vi "Find Workspace.vi"(8 "Error In":errorcluster, 10 "Control In":T2={"I-O.lvclass"=refnum, "Motion.lvclass"=refnum, "Dispenser.lvclass"=refnum}, 11 "Workspace In":refnum<class "Fixture.lvclass">) -> (0 "Error Out":errorcluster, 1 "Workspace Out":T1, 2 "Control Out":T2, 3 "Workspace Out":refnum<class "Fixture.lvclass">)   [LabVIEW 2016, in "Fixture.lvclass"]
uses:
  Fixture.lvclass
  Controller/Controllers.ctl
  Controller/I-O/I-O.lvclass
  Controller/Motion/A3200/A3200.lvclass
  Controller/Dispenser/Dispenser.lvclass
  Controller/Motion/Motion.lvclass
  Workspace.ctl
  Fixture.lvclass/Fixture.ctl
  Controller/Controller.lvclass
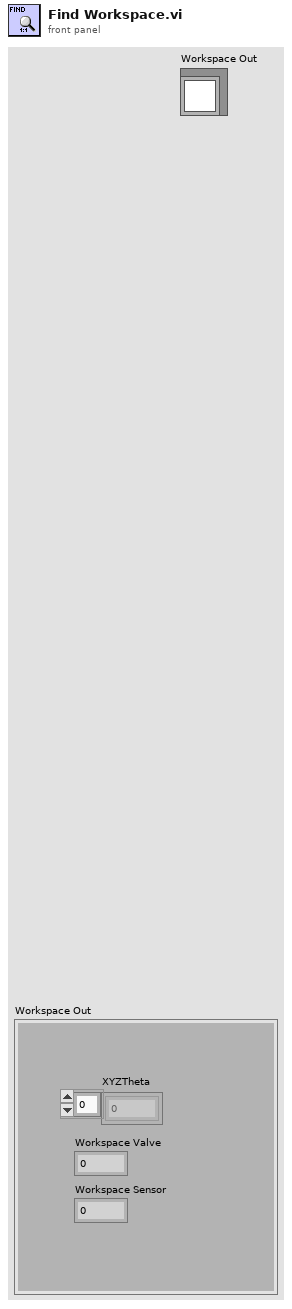
[diagram p1: front panel]
types:
  T1 = typedef "Fixture.lvclass/Workspace.ctl" = cluster{"XYZTheta":dbl[], "Workspace Valve":i32, "Workspace Sensor":i32}
  T2 = typedef "Controller.lvclass/Controllers.ctl" = cluster{"I-O.lvclass":refnum<class "I-O.lvclass">, "Motion.lvclass":refnum<class "Motion.lvclass">, "Dispenser.lvclass":refnum<class "Dispenser.lvclass">}
  T3 = typedef "I-O.lvclass/Pin Map.ctl" = cluster{"Region Valves":i32[], "Extra Valves":dbl[][][], "Tool Primary Valve":i32, "Tool Secondary Valve":i32, "Region Sensors":i32[], "Extra Sensors":dbl[][][], "Tool Primary Sensor":dbl, "Tool Secondary Sensor":dbl, "Compression Sensor":dbl, "5V":i32}
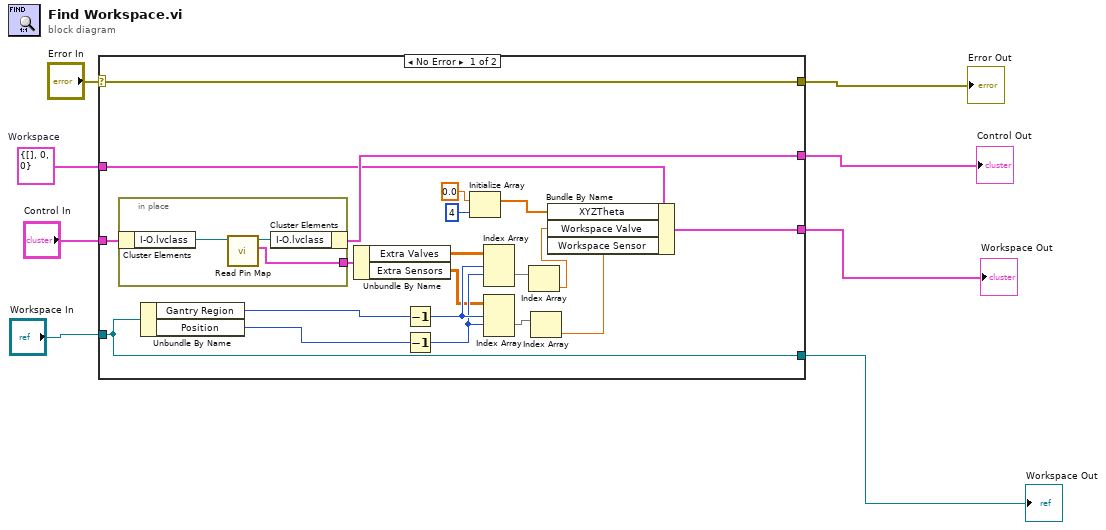
[diagram p0: block diagram]
diagram:
  w4 = T1 {"XYZTheta"=[], "Workspace Valve"=0, "Workspace Sensor"=0}  # Workspace
  n1 = case shown="No Error" "Error In" {
    selector: "Error In" -> [w28 w35]
    tunnel: [w28 w35] -> w7
    tunnel: [w23 w34] -> w5
    tunnel: "Workspace In" -> [w23 w34]
    tunnel: w4 -> [w19 w33]
    tunnel: [w21 w33] -> w3
    tunnel: "Control In" -> [w27 w32]
    tunnel: [w26 w32] -> w1
    frame No Error {
      n2 = in-place {
        in-place-border: [w29] -> w22
        n3 = in-place-cluster #1(w27) -> ("I-O.lvclass"=w31:refnum<class "I-O.lvclass">)
        n4 = call-dynamic "Read Pin Map.vi"("I-O in"=w31) -> ("Pin Map 2"=w29:T3, "I-O out"=w30:refnum<class "I-O.lvclass">)  [unwired: 8 in, 1 out]
        n5 = in-place-cluster #1("I-O.lvclass"=w30) -> (w26:T2)
      }
      n6 = Unbundle By Name(w23) -> ("Gantry Region"=w18:i32, "Position"=w16:i32)
      n7 = Unbundle By Name(w22) -> ("Extra Valves"=w14:dbl[][][], "Extra Sensors"=w13:dbl[][][])
      n8 = Decrement(x=w18) -> (x-1=w17:i32)
      n9 = Decrement(x=w16) -> (x-1=w15:i32)
      n10 = Initialize Array(0.0 ("element"), 4 ("dimension size")) -> (w20:dbl[])
      n11 = Index Array(array=w14, index (dim 0)=w17, index (dim 1)=w15) -> (element=w12:dbl[])  [unwired: 1 in]
      n12 = Index Array(array=w13, index (dim 0)=w17, index (dim 1)=w15) -> (element=w10:dbl[])  [unwired: 1 in]
      n13 = Index Array(array=w12) -> (element=w11:dbl)  [unwired: 1 in]
      n14 = Index Array(array=w10) -> (element=w9:dbl)  [unwired: 1 in]
      n15 = Bundle By Name(cluster=w19, "XYZTheta"=w20, "Workspace Valve"=w11, "Workspace Sensor"=w9) -> (w21:T1)
    }
    frame Error {
    }
  }
  "Error Out" <- w7
  "Workspace Out" <- w5
  "Control Out" <- w1
  "Workspace Out" <- w3
